vi "I2C_Write.vi"(8 "DataLow":u8=231 format="%x", 9 "DataUp":u8=1 format="%x", 10 "Reg":u8=4 format="%x", 11 "Device":u8=186 format="%x") -> (1 "ArrayLow":u64=2303591314090256358, 3 "ArrayUp":u64=1534)   [LabVIEW 2013]
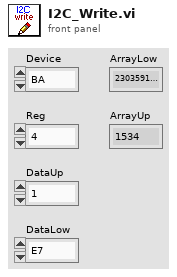
[diagram p1: front panel]
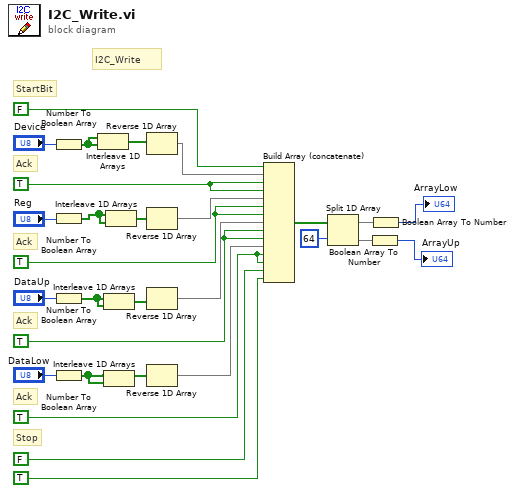
[diagram p0: block diagram]
diagram:
  w13 = TRUE
  w10 = TRUE
  w7 = TRUE
  w4 = TRUE
  # "Stop"
  # "Ack"
  # "Ack"
  # "Ack"
  # "Ack"
  # "StartBit"
  # "I2C_Write"
  n1 = Number To Boolean Array(number="Device") -> (Boolean array=w16:bool[])
  n2 = Number To Boolean Array(number="Reg") -> (Boolean array=w22:bool[])
  n3 = Number To Boolean Array(number="DataUp") -> (Boolean array=w21:bool[])
  n4 = Number To Boolean Array(number="DataLow") -> (Boolean array=w23:bool[])
  n5 = Interleave 1D Arrays(w16, w16) -> (w17:bool[])
  n6 = Interleave 1D Arrays(w21, w21) -> (w20:bool[])
  n7 = Interleave 1D Arrays(w23, w23) -> (w18:bool[])
  n8 = Interleave 1D Arrays(w22, w22) -> (w19:bool[])
  n9 = Reverse 1D Array(array=w17) -> (reversed array=w2:bool[])
  n10 = Reverse 1D Array(array=w19) -> (reversed array=w5:bool[])
  n11 = Reverse 1D Array(array=w20) -> (reversed array=w9:bool[])
  n12 = Reverse 1D Array(array=w18) -> (reversed array=w11:bool[])
  n13 = Build Array (concatenate)(FALSE, w2, w4, w4, w5, w7, w7, w9, w10, w10, w11, w13, w13, FALSE, TRUE) -> (w25:bool[])
  n14 = Split 1D Array(array=w25, index=u64 64) -> (first subarray=w26:bool[], second subarray=w27:bool[])
  n15 = Boolean Array To Number(Boolean array=w27) -> (number=→"ArrayUp":u64)
  n16 = Boolean Array To Number(Boolean array=w26) -> (number=→"ArrayLow":u64)
